vi "실습 2-7 불리언연산.vi"() -> ()   [LabVIEW 2014]
panel:
  in  "A 2":bool=TRUE
  in  "B 2":bool
  in  "C 2":bool
  out "D 2":bool=TRUE
  out "D":bool=TRUE
  in  "C":bool
  in  "B":bool
  in  "A":bool=TRUE
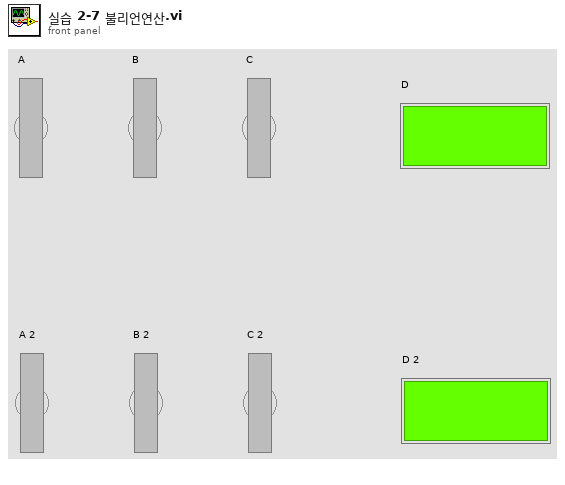
[diagram p1: front panel]
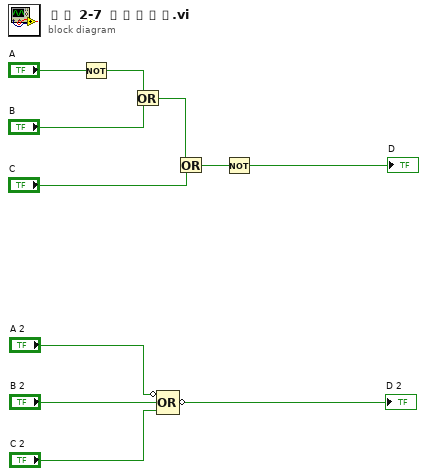
[diagram p0: block diagram]
diagram:
  n1 = Not(x="A") -> (.not. x?=w10:bool)
  n2 = Or(x=w10, y="B") -> (x .or. y?=w8:bool)
  n3 = Compound Arithmetic op=OR(invert "A 2", "B 2", "C 2") -> (invert →"D 2":bool)
  n4 = Or(x=w8, y="C") -> (x .or. y?=w6:bool)
  n5 = Not(x=w6) -> (.not. x?=→"D":bool)
